vi "load tdms image from fast acquisition app.vi"(11 "file path":path) -> (3 "Intensity Graph":u16[][](graph))   [LabVIEW 2020]
panel:
  out "number images":i32
  out "channel name out":string
  out "data 3":i32
  out "property names":string[](array[string])
  out "property values":variant[](array[variant])
  out "channel names":string[](array[string])
  out "found 2":bool
  out "found":bool
  out "width":i32
  out "size(s)":i32
  out "time to read":u32
  out "data":u16[](array[numeric])
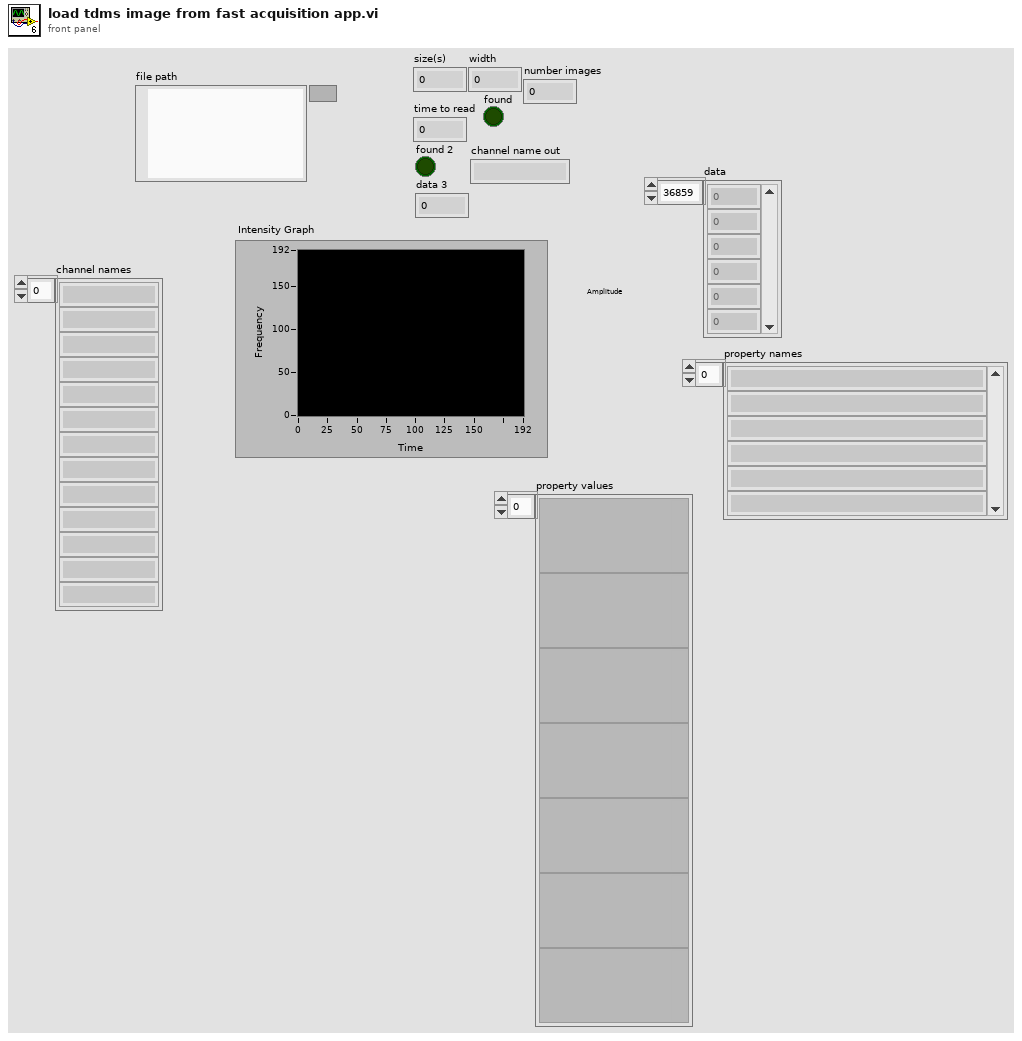
[diagram p1: front panel]
types:
  T1 = enum16{"open", "open or create", "create or replace", "create", "open (read-only)"}
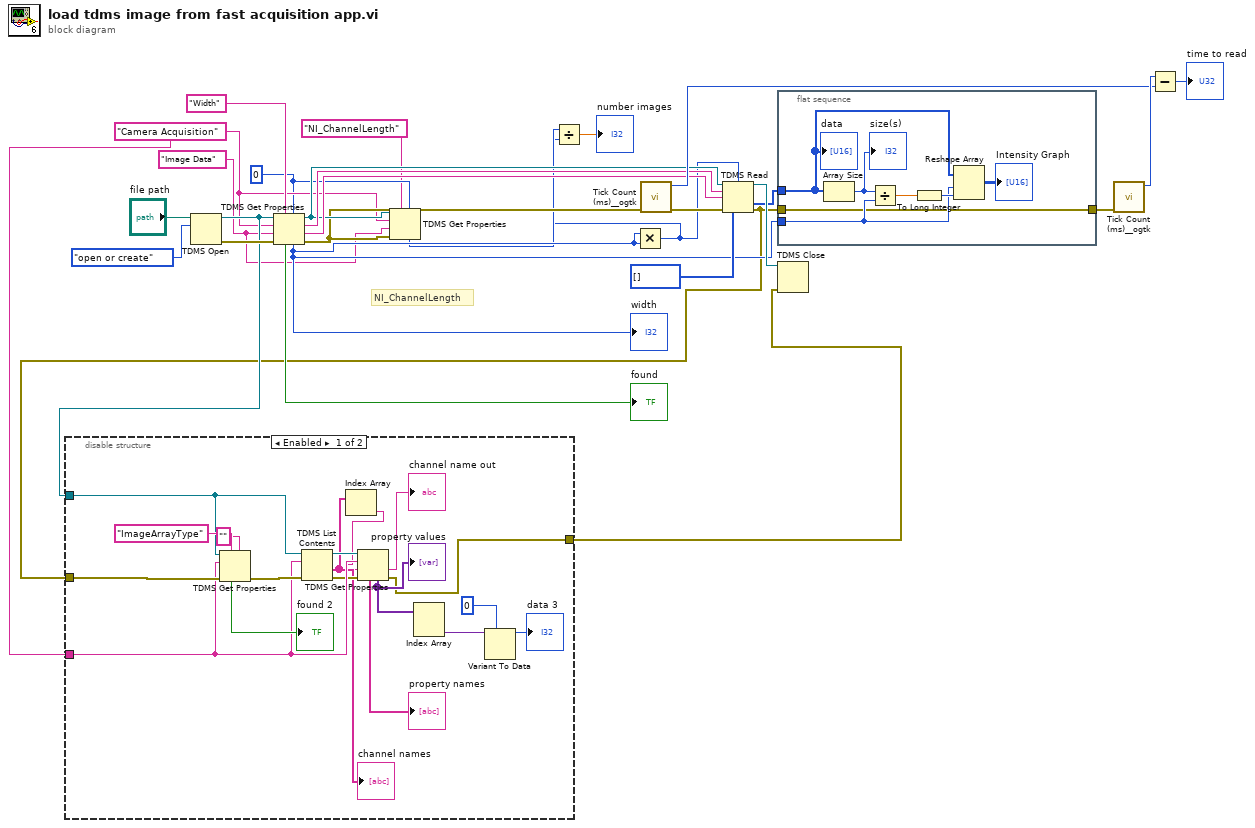
[diagram p0: block diagram]
diagram:
  w5 = 0 ("x")
  w7 = "Camera Acquisition" ("group name in")
  w6 = "Image Data" ("channel name(s) in")
  # "NI_ChannelLength"
  n1 = TDMS Open(10:T1."open or create" ("operation (0:open)"), 11:"file path") -> (0:w20:errorcluster, 3:w12:refnum<k34>)  [unwired: 5 in]
  n2 = TDMS Get Properties(5:w5, 7:"Width", 8:w20, 9:w6, 10:w7, 11:w12) -> (0:w8:errorcluster, 1:w13:string, 2:w14:string, 3:w9:refnum<k34>, 4:w15:i32, 6:→"found":bool)
  "width" <- w15
  n3 = TDMS Get Properties(5:w5, 7:"NI_ChannelLength" ("property name"), 8:w8, 9:w6, 10:w7, 11:w9) -> (4:w3:i32)  [unwired: 5 out]
  n4 = Multiply(x=w15, y=w15) -> (x*y=w2:i32)
  n5 = Divide(x=w3, y=w2) -> (x/y=→"number images":dbl)
  n6 = call <userlib>:"Tick Count (ms)__ogtk.vi"("error in (no error)"=w8) -> ("error out"=w26:errorcluster, "millisecond timer value"=w24:u32)  [unwired: 9 in]
  n7 = TDMS Read(0:w9, 2:w2, 5:w14, 7:w13, 11:w26, 12:u16[] [] ("output array")) -> (4:w23:refnum<k34>, 10:w18:u16[], 15:w11:errorcluster)  [unwired: 2 in, 3 out]
  n8 = disable-structure shown="Enabled" {
    disable-tunnel: w11 -> [w45 _]
    disable-tunnel: w12 -> [w42 _]
    disable-tunnel: [w33 _] -> w10
    disable-tunnel: w7 -> [w32 _]
    frame Enabled {
      n9 = TDMS Get Properties(5:"" ("data type"), 7:"ImageArrayType", 8:w45, 10:w32, 11:w42) -> (0:w41:errorcluster, 6:→"found 2":bool)  [unwired: 1 in, 4 out]
      n10 = TDMS List Contents(4:w41, 6:w32, 7:w42) -> (0:w31:errorcluster, 1:w30:string[], 3:w40:refnum<k34>)  [unwired: 1 out]
      "channel names" <- w30
      n11 = Index Array(array=w30) -> (element=w29:string)  [unwired: 1 in]
      n12 = TDMS Get Properties(8:w31, 9:w29, 10:w32, 11:w40) -> (0:w33:errorcluster, 1:→"channel name out":string, 4:w38:variant[], 6:→"property names":string[])  [unwired: 2 in, 2 out]
      "property values" <- w38
      n13 = Index Array(array=w38) -> (element #2=w34:variant)  [unwired: 2 in, 1 out]
      n14 = Variant To Data(type=0, Variant=w34) -> (data=→"data 3":i32)  [unwired: 1 in, 1 out]
    }
    frame Disabled {
    }
  }
  n15 = flat-sequence {
    tunnel: w18 -> [w53]
    tunnel: w15 -> [w48]
    tunnel: w11 -> [w47]
    tunnel: [w47] -> w16
    frame #0 {
      n16 = Array Size(array=w53) -> (size(s)=w52:i32)
      "size(s)" <- w52
      n17 = Divide(x=w52, y=w48) -> (x/y=w51:dbl)
      n18 = To Long Integer(number=w51) -> (32bit integer=w50:i32)
      n19 = Reshape Array(w53, w48, w50) -> (→"Intensity Graph":u16[][])
      "data" <- w53
    }
  }
  n20 = TDMS Close(8:w10, 11:w23) -> ()  [unwired: 2 out]
  n21 = call <userlib>:"Tick Count (ms)__ogtk.vi"("error in (no error)"=w16) -> ("millisecond timer value"=w25:u32)  [unwired: 9 in, 1 out]
  n22 = Subtract(x=w25, y=w24) -> (x-y=→"time to read":u32)
